vi "INIT.vi"(8 "error in (no error)":errorcluster, 11 "DAQmxTaksContainer_Emulate in":refnum<class "DAQmxTaksContainer_Emulate.lvclass">) -> (0 "error out":errorcluster, 3 "DAQmxTaksContainer_Emulate out":refnum<class "DAQmxTaksContainer_Emulate.lvclass">)   [LabVIEW 2018, in "DAQmxTaksContainer_Emulate.lvclass"]
uses:
  DAQmxTaksContainer_Emulate.lvclass
  C:/Users/Sergey Denisov/Documents/REPS/TRANCON/Classes/DAQmxTasks/DAQmxTaskContainer_General/DAQmxTaksContainer_General.lvclass
  C:/Users/Sergey Denisov/Documents/REPS/TRANCON/Classes/GeneralFunctionality/GeneralFunctionality.lvclass
  dependecies/ControlsVIs/Clusters-def/SERVER-Commands.ctl
  dependecies/ControlsVIs/Clusters-def/Message types.ctl
  DAQmxTaskContainer_General/DAQmxTaksContainer_General.lvclass/DAQmxTaksContainer_General.ctl
  DAQmxTaskContainer_General/DAQmxTaksContainer_General.lvclass
  DAQmxTask.lvclass
  Control/Control-Server/Control-Server.lvclass
  Message/Message.lvclass
  GeneralFunctionality/GeneralFunctionality.lvclass
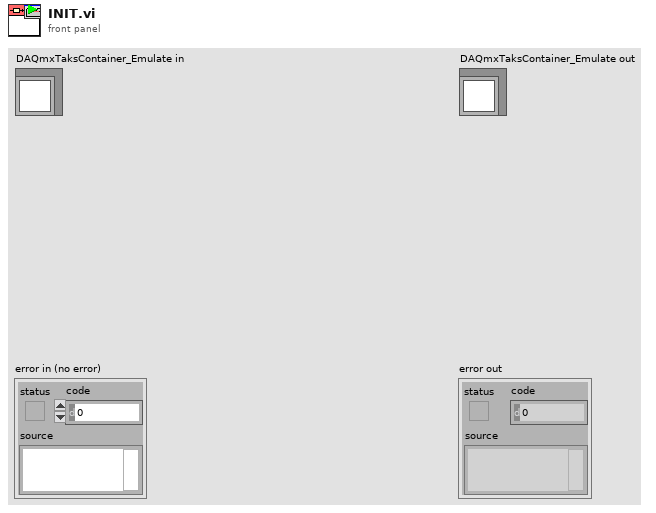
[diagram p1: front panel]
types:
  T1 = typedef "Message types.ctl" = string
  T2 = typedef "Control-Server.lvclass/SERVER-Commands.ctl" = string
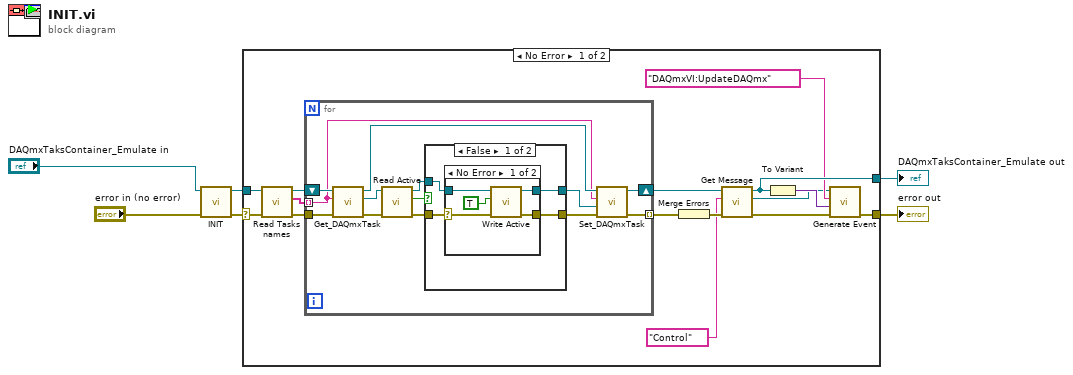
[diagram p0: block diagram]
diagram:
  n1 = call-parent "INIT.vi"("error in (no error)"="error in (no error)", "DAQmxTaksContainer_General in"="DAQmxTaksContainer_Emulate in") -> ("error out"=w1:errorcluster, "DAQmxTaksContainer_General out"=w2:refnum<class "DAQmxTaksContainer_Emulate.lvclass">)  [unwired: 8 in]
  n2 = case shown="No Error" w1 {
    selector: w1 -> [w7 w49]
    tunnel: [w17 w49] -> w5
    tunnel: [w19 w48] -> w6
    tunnel: w2 -> [w8 w48]
    frame No Error {
      n3 = call "Read Tasks names.vi"("error in (no error)"=w7, "DAQmxTaksContainer_General in"=w8) -> ("error out"=w12:errorcluster, "Tasks names"=w10:string[], "DAQmxTaksContainer_General out"=w11:refnum<class "DAQmxTaksContainer_Emulate.lvclass">)  [unwired: 7 in]
      n4 = for {
        tunnel: w10 -> [w26] mode=indexing
        tunnel: w12 -> [w30]
        tunnel: [w25] -> w21 mode=indexing
        shift-right: [w23] -> w18
        shift-left: w11 -> [w31]
        n5 = call "Get_DAQmxTask.vi"("error in (no error)"=w30, "Task name"=w26, "DAQmxTaksContainer_General in"=w31) -> ("error out"=w28:errorcluster, "DAQmx Task"=w29:refnum<class "DAQmxTask.lvclass">, "DAQmxTaksContainer_General out"=w27:refnum<class "DAQmxTaksContainer_Emulate.lvclass">)  [unwired: 6 in]
        n6 = call-dynamic "Read Active.vi"("error in (no error)"=w28, "DAQmxTask in"=w29) -> ("error out"=w32:errorcluster, "Active?"=w34:bool, "DAQmxTask out"=w33:refnum<class "DAQmxTask.lvclass">)  [unwired: 7 in]
        n7 = case shown="False" w34 {
          tunnel: w33 -> [w36 w47]
          tunnel: w32 -> [w35 w46]
          tunnel: [w38 w46] -> w24
          tunnel: [w37 w47] -> w22
          frame False {
            n8 = case shown="No Error" w35 {
              selector: w35 -> [w43 w44]
              tunnel: [w41 w44] -> w38
              tunnel: [w40 w45] -> w37
              tunnel: w36 -> [w39 w45]
              frame No Error {
                n9 = call-dynamic "Write Active.vi"("error in (no error)"=w43, "Active?"=TRUE, "DAQmxTask in"=w39) -> ("error out"=w41:errorcluster, "DAQmxTask out"=w40:refnum<class "DAQmxTask.lvclass">)  [unwired: 7 in]
              }
              frame Error {
              }
            }
          }
          frame True {
          }
        }
        n10 = call "Set_DAQmxTask.vi"("error in (no error)"=w24, "DAQmxTask"=w22, "Task name"=w26, "DAQmxTaksContainer_General in"=w27) -> ("error out"=w25:errorcluster, "DAQmxTaksContainer_General out"=w23:refnum<class "DAQmxTaksContainer_Emulate.lvclass">)  [unwired: 6 in]
      }
      n11 = Merge Errors(w21) -> (w20:errorcluster)
      n12 = call "Get Message.vi"("error in (no error)"=w20, "Message type"=T1 "Control", "GeneralFunctionality en entrée"=w18) -> ("error out"=w13:errorcluster, "Message.lvclass"=w14:refnum<class "Message.lvclass">, "GeneralFunctionality en sortie"=w19:refnum<class "DAQmxTaksContainer_Emulate.lvclass">)  [unwired: 6 in]
      n13 = To Variant(anything=w19) -> (Variant=w15:variant)
      n14 = call "Generate Event.vi"("error in (no error)"=w13, "Data"=w15, "Command"=T2 "DAQmxVI:UpdateDAQmx", "Message en entrée"=w14) -> ("error out"=w17:errorcluster)  [unwired: 6 in, 1 out]
    }
    frame Error {
    }
  }
  "error out" <- w5
  "DAQmxTaksContainer_Emulate out" <- w6
